vi "Create.vi"(7 "HostName":string, 8 "error in (no error)":errorcluster, 9 "Artifact Days":i32, 10 "Notification":string, 11 "Project Name":string) -> (0 "error out":errorcluster, 3 "CI Project out":refnum<class "CI Project.lvclass">)   [LabVIEW 2014, in "CI Project.lvclass"]
uses:
  CI Project.lvclass
  CI Project.lvclass/CI Project.ctl
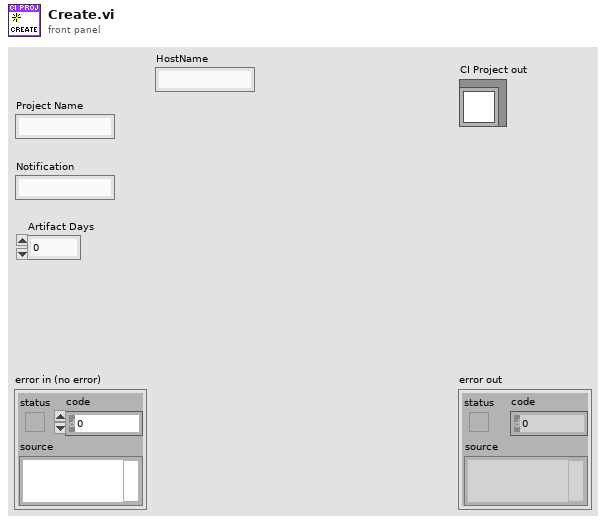
[diagram p1: front panel]
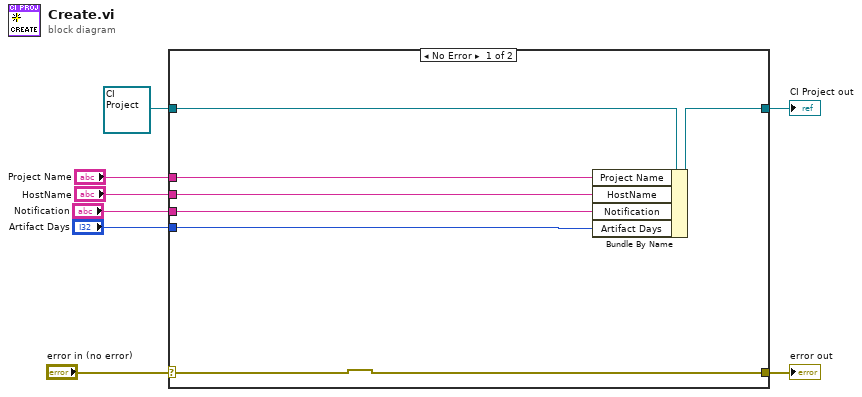
[diagram p0: block diagram]
diagram:
  n1 = case shown="No Error" "error in (no error)" {
    selector: "error in (no error)" -> [w9 w17]
    tunnel: [w9 w17] -> w7
    tunnel: [w14 w16] -> w5
    tunnel: refnum<class "CI Project.lvclass"> refnum ("CI Project in") -> [w15 w16]
    tunnel: "Project Name" -> [w13 _]
    tunnel: "HostName" -> [w12 _]
    tunnel: "Notification" -> [w11 _]
    tunnel: "Artifact Days" -> [w10 _]
    frame No Error {
      n2 = Bundle By Name(cluster=w15, "Project Name"=w13, "HostName"=w12, "Notification"=w11, "Artifact Days"=w10) -> (w14:refnum<class "CI Project.lvclass">)
    }
    frame Error {
    }
  }
  "error out" <- w7
  "CI Project out" <- w5
